vi "Simple Beep.vi"   [LabVIEW 2019]
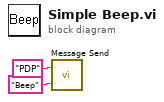
[diagram p0: block diagram]
diagram:
  n1 = call "Message Send.vi"("Message"="Beep", "Destination"="PDP") -> ()
